vi "Conf EZ.vi"(0 "VISA Resource Name":refnum<visa-resource-name>, 1 "Voltage/Freq/Period Conf":T2={"Range (5:Auto)"=enum."Auto", "Resolution (5:Default)"=enum."Default"}, 2 "Current Conf":T4={"Range (3:Auto)"=enum."Auto", "Resolution (3:Least)"=enum."Least"}, 3 "Resistance Conf":T3={"Range (7:Auto)"=enum."Auto", "Resolution (5:Default)"=enum."Default"}, 5 "Channel List(empty)":string, 7 "Set/Check (F:Set)":bool, 9 "Measurement (1:DC Volt)":T5(ring)=enum."DC Voltage", 11 "error in (no error)":errorcluster, 12 "Temperature Conf":T1={"Transducer Type (0:TC)"=enum."Thermocouple", "Thermocouple Type (8:Last)"=enum."Default (Last)", "Thermistor Type (3: Last)"=enum."Default (Last)", "RTD Type (2:Last)"=enum."Default (Last)"}, 13 "Digital (0:Byte)":u16(ring) items=["Byte"], 14 "Totalizer (0:Read)":enum16{"Read", "Read and Reset"}(ring)) -> (4 "VISA Resource Name Out":refnum<visa-resource-name>, 8 "Configuration?":string, 15 "error out":errorcluster)   [LabVIEW 2012, in "Agilent 34970.lvlib"]
doc: "This VI lets you configure the instrument for simple voltage, current, resistance, temperature, freq/period and, digital/totalizer measurements as well as setting up the scan list. Looking at the block diagram of \"HP34970A Advanced Scan Example.vi\", this VI replaces the specific measurment configuration commands (e.g. Conf Voltage) as well as the Conf Scan List VI. The trigger and read VIs are still needed to take a measurement. For more information on the different ways to take a measurment, refer to the context help and block diagram of the \"HP34970A Advanced Scan Example.vi\".\n\n* Note * There was a bug in the old driver giving the option to read a word from the digital port. This is not possible with the CONF command. To read a word, according to the documentation, put both digital input channels in the same scan list. The readings will be taken simultaneously and given the same timestamp."
uses:
  <instrlib>/Agilent 34970/Agilent 34970.lvlib
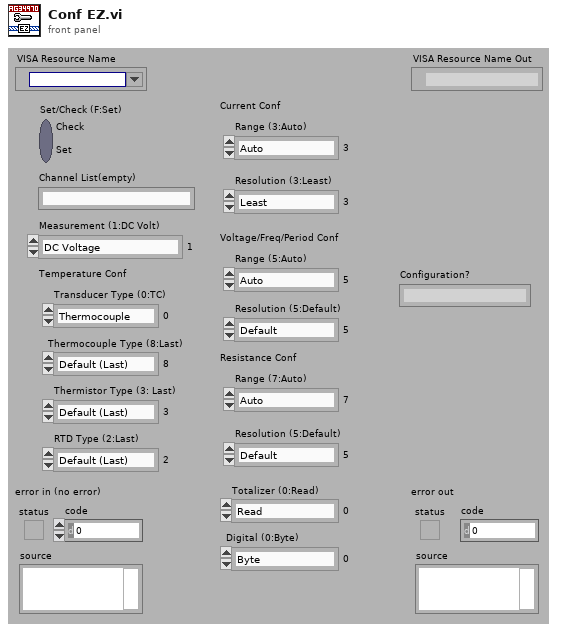
[diagram p1: front panel]
types:
  T1 = cluster{"Transducer Type (0:TC)":enum16{"Thermocouple", "Thermistor", "RTD", "4-Wire RTD", "Default (Last)"}, "Thermocouple Type (8:Last)":enum16{"B", "E", "J", "K", "N", "R", "S", "T", "Default (Last)"}, "Thermistor Type (3: Last)":enum16{"2252", "5000", "10000", "Default (Last)"}, "RTD Type (2:Last)":enum16{"85", "91", "Default (Last)"}}
  T2 = cluster{"Range (5:Auto)":enum16{"100 mV", "1 V", "10 V", "100 V", "300 V", "Auto", "Minimum", "Maximum"}, "Resolution (5:Default)":enum16{"4 1/2", "5 1/2", "6 1/2", "Least", "Highest", "Default"}}
  T3 = cluster{"Range (7:Auto)":enum16{"100 Ohm", "1 kOhm", "10 kOhm", "100 kOhm", "1 MOhm", "10 MOhm", "100 MOhm", "Auto", "Minimum", "Maximum"}, "Resolution (5:Default)":enum16{"4 1/2", "5 1/2", "6 1/2", "Least", "Highest", "Default"}}
  T4 = cluster{"Range (3:Auto)":enum16{"10 mA", "100 mA", "1 A", "Auto", "Minimum", "Maximum"}, "Resolution (3:Least)":enum16{"4 1/2", "5 1/2", "6 1/2", "Least", "Highest", "Default"}}
  T5 = enum16{"Temperature", "DC Voltage", "AC Voltage", "DC Current", "AC Current", "Resistance", "4-Wire Resistance", "Frequency", "Period", "Digital", "Totalizer"}
  T6 = enum16{"Thermocouple", "Thermistor", "RTD", "4-Wire RTD", "Default (Last)"}
  T7 = enum16{"B", "E", "J", "K", "N", "R", "S", "T", "Default (Last)"}
  T8 = enum16{"2252", "5000", "10000", "Default (Last)"}
  T9 = enum16{"100 mV", "1 V", "10 V", "100 V", "300 V", "Auto", "Minimum", "Maximum"}
  T10 = enum16{"4 1/2", "5 1/2", "6 1/2", "Least", "Highest", "Default"}
  T11 = enum16{"100 Ohm", "1 kOhm", "10 kOhm", "100 kOhm", "1 MOhm", "10 MOhm", "100 MOhm", "Auto", "Minimum", "Maximum"}
  T12 = enum16{"10 mA", "100 mA", "1 A", "Auto", "Minimum", "Maximum"}
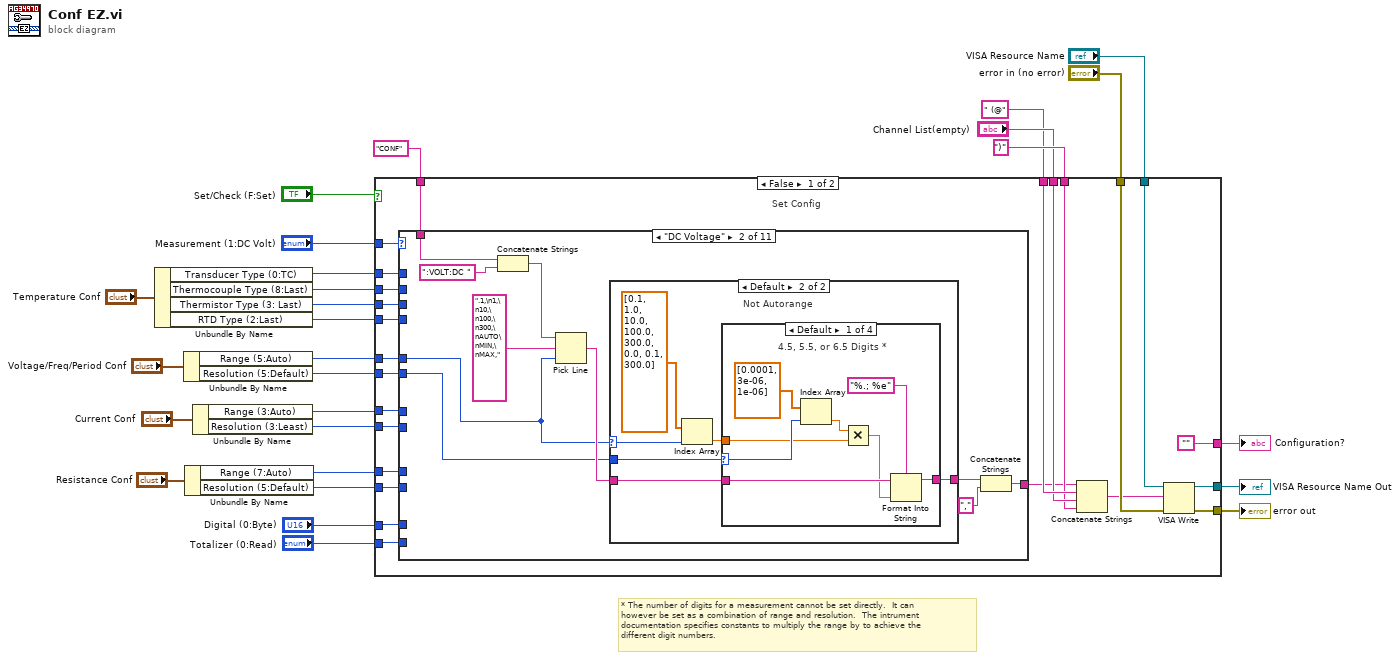
[diagram p0: block diagram]
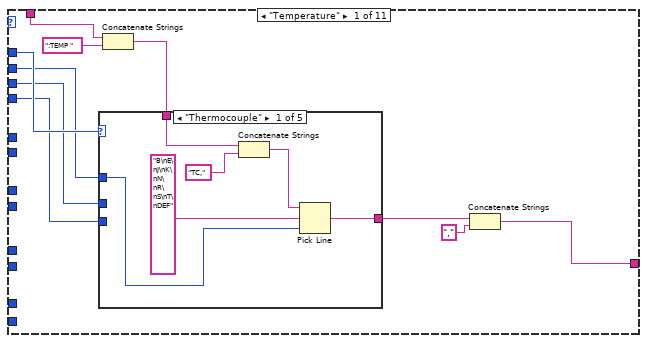
[diagram p2: hidden frame]
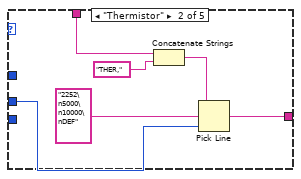
[diagram p3: hidden frame]
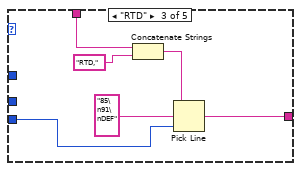
[diagram p4: hidden frame]
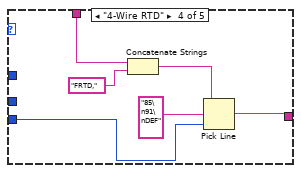
[diagram p5: hidden frame]
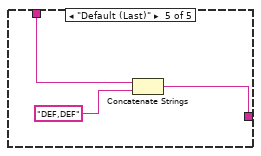
[diagram p6: hidden frame]
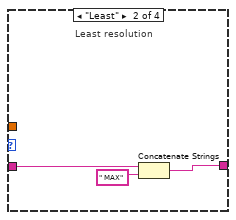
[diagram p8: hidden frame]
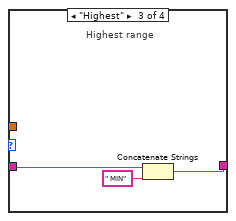
[diagram p9: hidden frame]
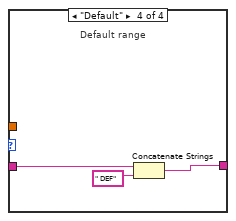
[diagram p10: hidden frame]
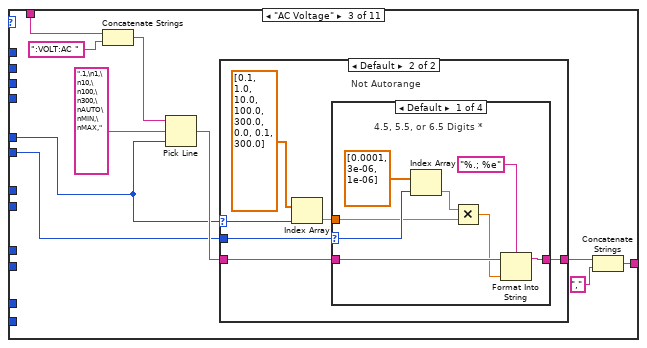
[diagram p11: hidden frame]
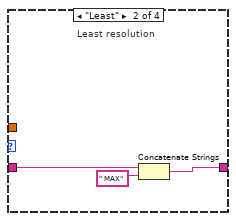
[diagram p13: hidden frame]
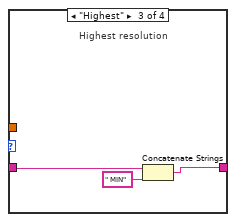
[diagram p14: hidden frame]
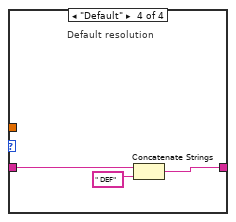
[diagram p15: hidden frame]
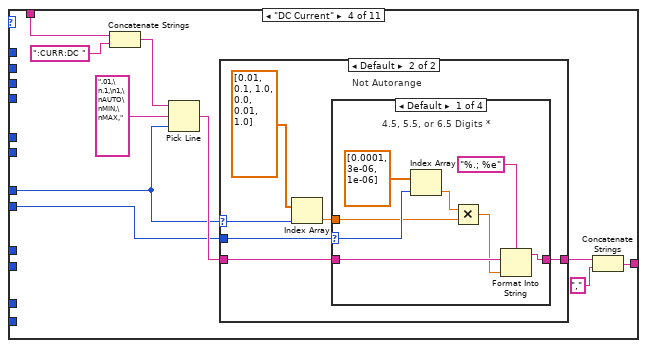
[diagram p16: hidden frame]
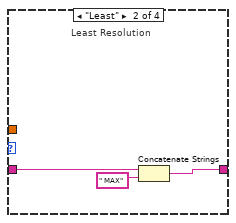
[diagram p18: hidden frame]
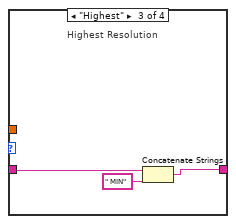
[diagram p19: hidden frame]
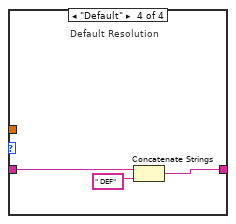
[diagram p20: hidden frame]
diagram:
  # "* The number of digits for a measurement cannot be set directly.  It can\nhowever be set as a combination of range and resolution.  The intrument\ndocumentation specifies constants to multiply the range by to achieve the\ndifferent digit numbers."
  n1 = Unbundle By Name("Temperature Conf") -> ("Transducer Type (0:TC)"=w17:T6, "Thermocouple Type (8:Last)"=w16:T7, "Thermistor Type (3: Last)"=w15:T8, "RTD Type (2:Last)"=w14:enum16{"85", "91", "Default (Last)"})
  n2 = Unbundle By Name("Voltage/Freq/Period Conf") -> ("Range (5:Auto)"=w12:T9, "Resolution (5:Default)"=w11:T10)
  n3 = Unbundle By Name("Resistance Conf") -> ("Range (7:Auto)"=w6:T11, "Resolution (5:Default)"=w5:T10)
  n4 = Unbundle By Name("Current Conf") -> ("Range (3:Auto)"=w9:T12, "Resolution (3:Least)"=w8:T10)
  n5 = case shown="False" "Set/Check (F:Set)" {
    tunnel: " (@" -> [w51 w314]
    tunnel: "Channel List(empty)" -> [w50 w327]
    tunnel: ")" -> [w49 w326]
    tunnel: "Totalizer (0:Read)" -> [w48 _]
    tunnel: "Digital (0:Byte)" -> [w47 _]
    tunnel: w14 -> [w46 _]
    tunnel: w15 -> [w45 _]
    tunnel: w16 -> [w44 _]
    tunnel: w17 -> [w43 _]
    tunnel: "Measurement (1:DC Volt)" -> [w42 _]
    tunnel: "CONF" -> [w41 w325]
    tunnel: "VISA Resource Name" -> [w39 w323]
    tunnel: "error in (no error)" -> [w40 w322]
    tunnel: ["" w318] -> w19
    tunnel: [w38 w317] -> w4
    tunnel: [w37 w316] -> w3
    tunnel: w12 -> [w35 _]
    tunnel: w11 -> [w34 _]
    tunnel: w9 -> [w33 _]
    tunnel: w8 -> [w32 _]
    tunnel: w6 -> [w31 _]
    tunnel: w5 -> [w30 _]
    frame False {
      # "Set Config"
      n6 = case shown="\"DC Voltage\"" w42 {
        tunnel: w43 -> [w59 _ _ _ _ _ _ _ _ _ _]
        tunnel: w44 -> [w58 _ _ _ _ _ _ _ _ _ _]
        tunnel: w45 -> [w57 _ _ _ _ _ _ _ _ _ _]
        tunnel: w46 -> [w56 _ _ _ _ _ _ _ _ _ _]
        tunnel: w41 -> [w55 w97 w131 w165 w199 w233 w267 w297 w303 w307 w311]
        tunnel: w47 -> [_ _ _ _ _ _ _ _ _ _ _]
        tunnel: w48 -> [_ _ _ _ _ _ _ _ _ _ w312]
        tunnel: w35 -> [_ w92 w126 _ _ _ _ w294 w299 _ _]
        tunnel: w34 -> [_ w93 w127 _ _ _ _ _ _ _ _]
        tunnel: w33 -> [_ _ _ w161 w195 _ _ _ _ _ _]
        tunnel: w32 -> [_ _ _ w160 w194 _ _ _ _ _ _]
        tunnel: w31 -> [_ _ _ _ _ w229 w263 _ _ _ _]
        tunnel: w30 -> [_ _ _ _ _ w228 w262 _ _ _ _]
        tunnel: [w53 w90 w123 w158 w192 w226 w259 w293 w300 w306 w308] -> w29
        frame "Temperature" {
          n7 = Concatenate Strings(w55, ":TEMP ") -> (w60:string)
          n8 = case shown="\"Thermocouple\"" w59 {
            tunnel: w60 -> [w66 w69 w76 w81 w87]
            tunnel: [w63 w70 w75 w82 w86] -> w54
            tunnel: w58 -> [w62 _ _ _ _]
            tunnel: w57 -> [_ w68 _ _ _]
            tunnel: w56 -> [_ _ w74 w80 _]
            frame "Thermocouple" {
              n9 = Concatenate Strings(w66, "TC,") -> (w64:string)
              n10 = Pick Line(string ("")=w64, multi-line string="B\nE\nJ\nK\nN\nR\nS\nT\nDEF", line index=w62) -> (output string=w63:string)
            }
            frame "Thermistor" {
              n11 = Concatenate Strings(w69, "THER,") -> (w71:string)
              n12 = Pick Line(string ("")=w71, multi-line string="2252\n5000\n10000\nDEF", line index=w68) -> (output string=w70:string)
            }
            frame "RTD" {
              n13 = Concatenate Strings(w76, "RTD,") -> (w79:string)
              n14 = Pick Line(string ("")=w79, multi-line string="85\n91\nDEF", line index=w74) -> (output string=w75:string)
            }
            frame "4-Wire RTD" {
              n15 = Concatenate Strings(w81, "FRTD,") -> (w85:string)
              n16 = Pick Line(string ("")=w85, multi-line string="85\n91\nDEF", line index=w80) -> (output string=w82:string)
            }
            frame "Default (Last)" {
              n17 = Concatenate Strings(w87, "DEF,DEF") -> (w86:string)
            }
          }
          n18 = Concatenate Strings(w54, "," ("string")) -> (w53:string)
        }
        frame "DC Voltage" {
          n19 = Concatenate Strings(w97, ":VOLT:DC ") -> (w95:string)
          n20 = Pick Line(string ("")=w95, multi-line string=".1,\n1,\n10,\n100,\n300,\nAUTO\nMIN,\nMAX,", line index=w92) -> (output string=w94:string)
          n21 = case shown="Default" w92 {
            selector: w92 -> [_ w105]
            tunnel: [w99 w102] -> w91
            tunnel: w94 -> [w99 w101]
            tunnel: w93 -> [_ w103]
            frame "Auto" {
              # "Autorange"
            }
            frame Default {
              # "Not Autorange"
              n22 = Index Array(array=dbl[] [0.1, 1.0, 10.0, 100.0, 300.0, 0.0, 0.1, 300.0], index=w105) -> (element=w100:dbl)
              n23 = case shown="Default" w103 {
                selector: w103 -> [w112 _ _ _]
                tunnel: [w106 w116 w119 w120] -> w102
                tunnel: w101 -> [w109 w115 w117 w121]
                tunnel: w100 -> [w111 _ _ _]
                frame Default {
                  # "4.5, 5.5, or 6.5 Digits *"
                  n24 = Index Array(array=dbl[] [0.0001, 3e-06, 1e-06], index=w112) -> (element=w110:dbl)
                  n25 = Multiply(x=w110, y=w111) -> (x*y=w108:dbl)
                  n26 = Format Into String(format string="%.; %e", initial string=w109, w108) -> (resulting string=w106:string)  [unwired: 1 in, 1 out]
                }
                frame "Least" {
                  # "Least resolution"
                  n27 = Concatenate Strings(w115, " MAX" ("string")) -> (w116:string)
                }
                frame "Highest" {
                  # "Highest range"
                  n28 = Concatenate Strings(w117, " MIN" ("string")) -> (w119:string)
                }
                frame "Default" {
                  # "Default range"
                  n29 = Concatenate Strings(w121, " DEF" ("string")) -> (w120:string)
                }
              }
            }
          }
          n30 = Concatenate Strings(w91, "," ("string")) -> (w90:string)
        }
        frame "AC Voltage" {
          n31 = Concatenate Strings(w131, ":VOLT:AC ") -> (w129:string)
          n32 = Pick Line(string ("")=w129, multi-line string=".1,\n1,\n10,\n100,\n300,\nAUTO\nMIN,\nMAX,", line index=w126) -> (output string=w128:string)
          n33 = case shown="Default" w126 {
            selector: w126 -> [_ w139]
            tunnel: [w133 w136] -> w124
            tunnel: w128 -> [w133 w135]
            tunnel: w127 -> [_ w137]
            frame "Auto" {
              # "Autorange"
            }
            frame Default {
              # "Not Autorange"
              n34 = Index Array(array=dbl[] [0.1, 1.0, 10.0, 100.0, 300.0, 0.0, 0.1, 300.0], index=w139) -> (element=w134:dbl)
              n35 = case shown="Default" w137 {
                selector: w137 -> [w146 _ _ _]
                tunnel: [w140 w150 w153 w154] -> w136
                tunnel: w135 -> [w143 w149 w151 w155]
                tunnel: w134 -> [w145 _ _ _]
                frame Default {
                  # "4.5, 5.5, or 6.5 Digits *"
                  n36 = Index Array(array=dbl[] [0.0001, 3e-06, 1e-06], index=w146) -> (element=w144:dbl)
                  n37 = Multiply(x=w144, y=w145) -> (x*y=w142:dbl)
                  n38 = Format Into String(format string="%.; %e", initial string=w143, w142) -> (resulting string=w140:string)  [unwired: 1 in, 1 out]
                }
                frame "Least" {
                  # "Least resolution"
                  n39 = Concatenate Strings(w149, " MAX" ("string")) -> (w150:string)
                }
                frame "Highest" {
                  # "Highest resolution"
                  n40 = Concatenate Strings(w151, " MIN" ("string")) -> (w153:string)
                }
                frame "Default" {
                  # "Default resolution"
                  n41 = Concatenate Strings(w155, " DEF" ("string")) -> (w154:string)
                }
              }
            }
          }
          n42 = Concatenate Strings(w124, "," ("string")) -> (w123:string)
        }
        frame "DC Current" {
          n43 = Concatenate Strings(w165, ":CURR:DC ") -> (w163:string)
          n44 = Pick Line(string ("")=w163, multi-line string=".01,\n.1,\n1,\nAUTO\nMIN,\nMAX,", line index=w161) -> (output string=w162:string)
          n45 = case shown="Default" w161 {
            selector: w161 -> [_ w173]
            tunnel: [w167 w170] -> w157
            tunnel: w162 -> [w167 w169]
            tunnel: w160 -> [_ w171]
            frame "Auto" {
              # "Autorange"
            }
            frame Default {
              # "Not Autorange"
              n46 = Index Array(array=dbl[] [0.01, 0.1, 1.0, 0.0, 0.01, 1.0], index=w173) -> (element=w168:dbl)
              n47 = case shown="Default" w171 {
                selector: w171 -> [w180 _ _ _]
                tunnel: [w174 w184 w187 w188] -> w170
                tunnel: w169 -> [w177 w183 w185 w189]
                tunnel: w168 -> [w179 _ _ _]
                frame Default {
                  # "4.5, 5.5, or 6.5 Digits *"
                  n48 = Index Array(array=dbl[] [0.0001, 3e-06, 1e-06], index=w180) -> (element=w178:dbl)
                  n49 = Multiply(x=w178, y=w179) -> (x*y=w176:dbl)
                  n50 = Format Into String(format string="%.; %e", initial string=w177, w176) -> (resulting string=w174:string)  [unwired: 1 in, 1 out]
                }
                frame "Least" {
                  # "Least Resolution"
                  n51 = Concatenate Strings(w183, " MAX" ("string")) -> (w184:string)
                }
                frame "Highest" {
                  # "Highest Resolution"
                  n52 = Concatenate Strings(w185, " MIN" ("string")) -> (w187:string)
                }
                frame "Default" {
                  # "Default Resolution"
                  n53 = Concatenate Strings(w189, " DEF" ("string")) -> (w188:string)
                }
              }
            }
          }
          n54 = Concatenate Strings(w157, "," ("string")) -> (w158:string)
        }
        frame "AC Current" {
          n55 = Concatenate Strings(w199, ":CURR:AC ") -> (w197:string)
          n56 = Pick Line(string ("")=w197, multi-line string=".01,\n.1,\n1,\nAUTO\nMIN,\nMAX,", line index=w195) -> (output string=w196:string)
          n57 = case shown="Default" w195 {
            selector: w195 -> [_ w207]
            tunnel: [w201 w204] -> w191
            tunnel: w196 -> [w201 w203]
            tunnel: w194 -> [_ w205]
            frame "Auto" {
              # "Autorange"
            }
            frame Default {
              # "Not autorange"
              n58 = Index Array(array=dbl[] [0.01, 0.1, 1.0, 0.0, 0.01, 1.0], index=w207) -> (element=w202:dbl)
              n59 = case shown="\"Least\"" w205 {
                selector: w205 -> [w214 _ _ _]
                tunnel: [w208 w218 w221 w222] -> w204
                tunnel: w203 -> [w211 w217 w219 w223]
                tunnel: w202 -> [w213 _ _ _]
                frame Default {
                  # "4.5, 5.5, or 6.5 Digits *"
                  n60 = Index Array(array=dbl[] [0.0001, 3e-06, 1e-06], index=w214) -> (element=w212:dbl)
                  n61 = Multiply(x=w212, y=w213) -> (x*y=w210:dbl)
                  n62 = Format Into String(format string="%.; %e", initial string=w211, w210) -> (resulting string=w208:string)  [unwired: 1 in, 1 out]
                }
                frame "Least" {
                  # "Least Resolution"
                  n63 = Concatenate Strings(w217, " MAX" ("string")) -> (w218:string)
                }
                frame "Highest" {
                  # "Highest resolution"
                  n64 = Concatenate Strings(w219, " MIN" ("string")) -> (w221:string)
                }
                frame "Default" {
                  # "Default resolution"
                  n65 = Concatenate Strings(w223, " DEF" ("string")) -> (w222:string)
                }
              }
            }
          }
          n66 = Concatenate Strings(w191, "," ("string")) -> (w192:string)
        }
        frame "Resistance" {
          n67 = Concatenate Strings(w233, ":RES ") -> (w231:string)
          n68 = Pick Line(string ("")=w231, multi-line string="1e2,\n1e3,\n10e3,\n100e3,\n1e6,\n10e6,\n100e6,\nAUTO\nMIN,\nMAX,", line index=w229) -> (output string=w230:string)
          n69 = case shown="Default" w229 {
            selector: w229 -> [_ w241]
            tunnel: [w235 w238] -> w225
            tunnel: w230 -> [w235 w237]
            tunnel: w228 -> [_ w239]
            frame "Auto" {
              # "Autorange"
            }
            frame Default {
              # "Not Autorange"
              n70 = Index Array(array=dbl[] [100.0, 1000.0, 10000.0, 100000.0, 1000000.0, 10000000.0, 100000000.0, 0.0, 100.0, 100000000.0], index=w241) -> (element=w236:dbl)
              n71 = case shown="Default" w239 {
                selector: w239 -> [w248 _ _ _]
                tunnel: [w242 w252 w255 w256] -> w238
                tunnel: w237 -> [w245 w251 w253 w257]
                tunnel: w236 -> [w247 _ _ _]
                frame Default {
                  # "4.5, 5.5, or 6.5 Digits *"
                  n72 = Index Array(array=dbl[] [0.0001, 3e-06, 1e-06], index=w248) -> (element=w246:dbl)
                  n73 = Multiply(x=w246, y=w247) -> (x*y=w244:dbl)
                  n74 = Format Into String(format string="%.; %e", initial string=w245, w244) -> (resulting string=w242:string)  [unwired: 1 in, 1 out]
                }
                frame "Least" {
                  # "Least Resolution"
                  n75 = Concatenate Strings(w251, " MAX" ("string")) -> (w252:string)
                }
                frame "Highest" {
                  # "Highest Resolution"
                  n76 = Concatenate Strings(w253, " MIN" ("string")) -> (w255:string)
                }
                frame "Default" {
                  # "Default Resolution"
                  n77 = Concatenate Strings(w257, " DEF" ("string")) -> (w256:string)
                }
              }
            }
          }
          n78 = Concatenate Strings(w225, "," ("string")) -> (w226:string)
        }
        frame "4-Wire Resistance" {
          n79 = Concatenate Strings(w267, ":FRES ") -> (w265:string)
          n80 = Pick Line(string ("")=w265, multi-line string="1e2,\n1e3,\n10e3,\n100e3,\n1e6,\n10e6,\n100e6,\nAUTO\nMIN,\nMAX,", line index=w263) -> (output string=w264:string)
          n81 = case shown="Default" w263 {
            selector: w263 -> [_ w275]
            tunnel: [w269 w272] -> w260
            tunnel: w264 -> [w269 w271]
            tunnel: w262 -> [_ w273]
            frame "Auto" {
              # "Autorange"
            }
            frame Default {
              # "Not Autorange"
              n82 = Index Array(array=dbl[] [100.0, 1000.0, 10000.0, 100000.0, 1000000.0, 10000000.0, 100000000.0, 0.0, 100.0, 100000000.0], index=w275) -> (element=w270:dbl)
              n83 = case shown="Default" w273 {
                selector: w273 -> [w282 _ _ _]
                tunnel: [w276 w286 w289 w290] -> w272
                tunnel: w271 -> [w279 w285 w287 w291]
                tunnel: w270 -> [w281 _ _ _]
                frame Default {
                  # "4.5, 5.5, or 6.5 Digits *"
                  n84 = Index Array(array=dbl[] [0.0001, 3e-06, 1e-06], index=w282) -> (element=w280:dbl)
                  n85 = Multiply(x=w280, y=w281) -> (x*y=w278:dbl)
                  n86 = Format Into String(format string="%.; %e", initial string=w279, w278) -> (resulting string=w276:string)  [unwired: 1 in, 1 out]
                }
                frame "Least" {
                  # "Least Resolution"
                  n87 = Concatenate Strings(w285, " MAX" ("string")) -> (w286:string)
                }
                frame "Highest" {
                  # "Highest Resolution"
                  n88 = Concatenate Strings(w287, " MIN" ("string")) -> (w289:string)
                }
                frame "Default" {
                  # "Default Resolution"
                  n89 = Concatenate Strings(w291, " DEF" ("string")) -> (w290:string)
                }
              }
            }
          }
          n90 = Concatenate Strings(w260, "," ("string")) -> (w259:string)
        }
        frame "Frequency" {
          n91 = Concatenate Strings(w297, ":FREQ 20,") -> (w295:string)
          n92 = Pick Line(string ("")=w295, multi-line string=".1,\n1,\n10,\n100,\n300,\n\nMIN,\nMAX,", line index=w294) -> (output string=w293:string)
        }
        frame "Period" {
          n93 = Concatenate Strings(w303, ":PER .05") -> (w301:string)
          n94 = Pick Line(string ("")=w301, multi-line string=",.1,\n,1,\n,10,\n,100,\n,300,\n,\n,MIN,\n,MAX,", line index=w299) -> (output string=w300:string)
        }
        frame "Digital" {
          # "There was an bug in the old driver giving the option\nto read a word from the digital port.  This is not possible\nwith the CONF command.  To read a word, according to\nthe documentation, put both digital input channels in the\nsame scan list.  The readings will be taken simultaneously \nand given the same timestamp."
          n95 = Concatenate Strings(w307, ":DIG:BYTE " ("string")) -> (w306:string)
        }
        frame "Totalizer" {
          n96 = Pick Line(string ("")=w311, multi-line string=":TOT READ\n:TOT RRES", line index=w312) -> (output string=w310:string)
          n97 = Concatenate Strings(w310, "," ("string")) -> (w308:string)
        }
      }
      n98 = Concatenate Strings(w29, w51, w50, w49) -> (w28:string)
      n99 = VISA Write(VISA resource name=w39, write buffer=w28, error in (no error)=w40) -> (VISA resource name out=w38:refnum<visa-resource-name>, error out=w37:errorcluster)  [unwired: 1 out]
    }
    frame True {
      # "Check Config"
      n100 = Concatenate Strings(w325, "? ") -> (w324:string)
      n101 = Concatenate Strings(w324, w314, w327, w326) -> (w315:string)
      n102 = VISA Write(VISA resource name=w323, write buffer=w315, error in (no error)=w322) -> (VISA resource name out=w321:refnum<visa-resource-name>, error out=w320:errorcluster)  [unwired: 1 out]
      n103 = VISA Read(VISA resource name=w321, byte count=u32 100 ("byte count (0)"), error in (no error)=w320) -> (VISA resource name out=w317:refnum<visa-resource-name>, read buffer=w318:string, error out=w316:errorcluster)  [unwired: 1 out]
    }
  }
  "Configuration?" <- w19
  "error out" <- w3
  "VISA Resource Name Out" <- w4
